vi "wrapper.vi"() -> ()   [LabVIEW 2016]
uses:
  QSM-PC (String)/Library/QSM-PC (String).lvlib
panel:
  out "控件值:QSM-Main":variant
  out "cluster_from main":cluster{"State":string, "Data":variant}
  out "cluster_\nsend to main":cluster{"State":string, "Data":variant}
  out "command":string
  out "ReadLine":string
  out "main_controls":cluster{"Name":string, "Variant Data":variant}[](array[cluster])
  out "QSM - wrapper":refnum<queue>
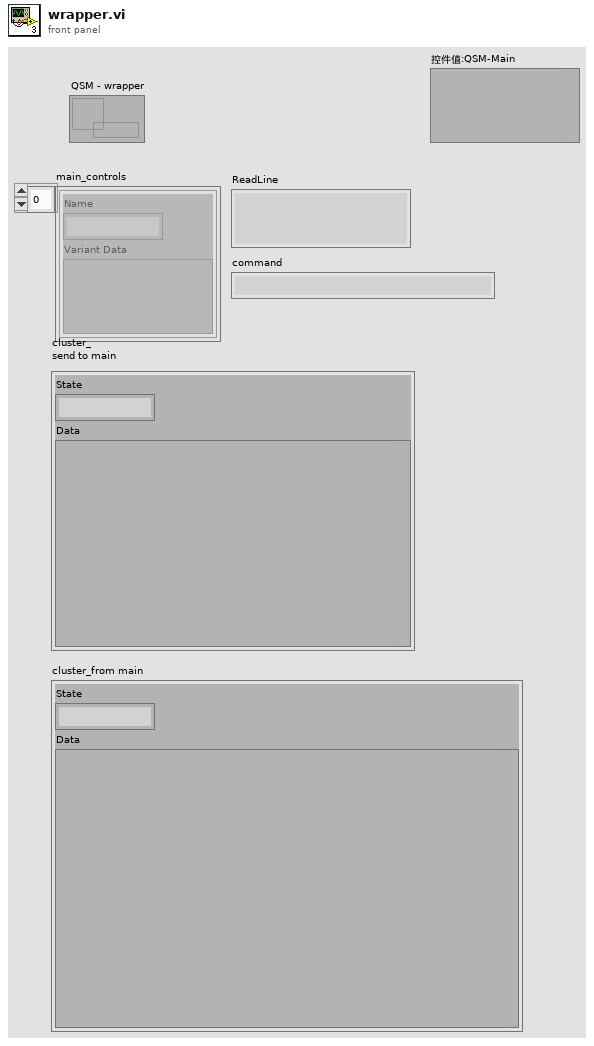
[diagram p1: front panel]
types:
  T1 = cluster{"app":string, "subject":string, "payload":cluster{"callback_msg":string}}
  T2 = cluster{"app":string, "subject":string, "payload":cluster{"callback_msg":dbl[][]}}
  T3 = cluster{"app":string, "subject":string, "payload":cluster{"time":string}}
  T4 = cluster{"app":string, "command":string, "payload":string}
  T5 = cluster{"app":string, "command":string, "payload":dbl}
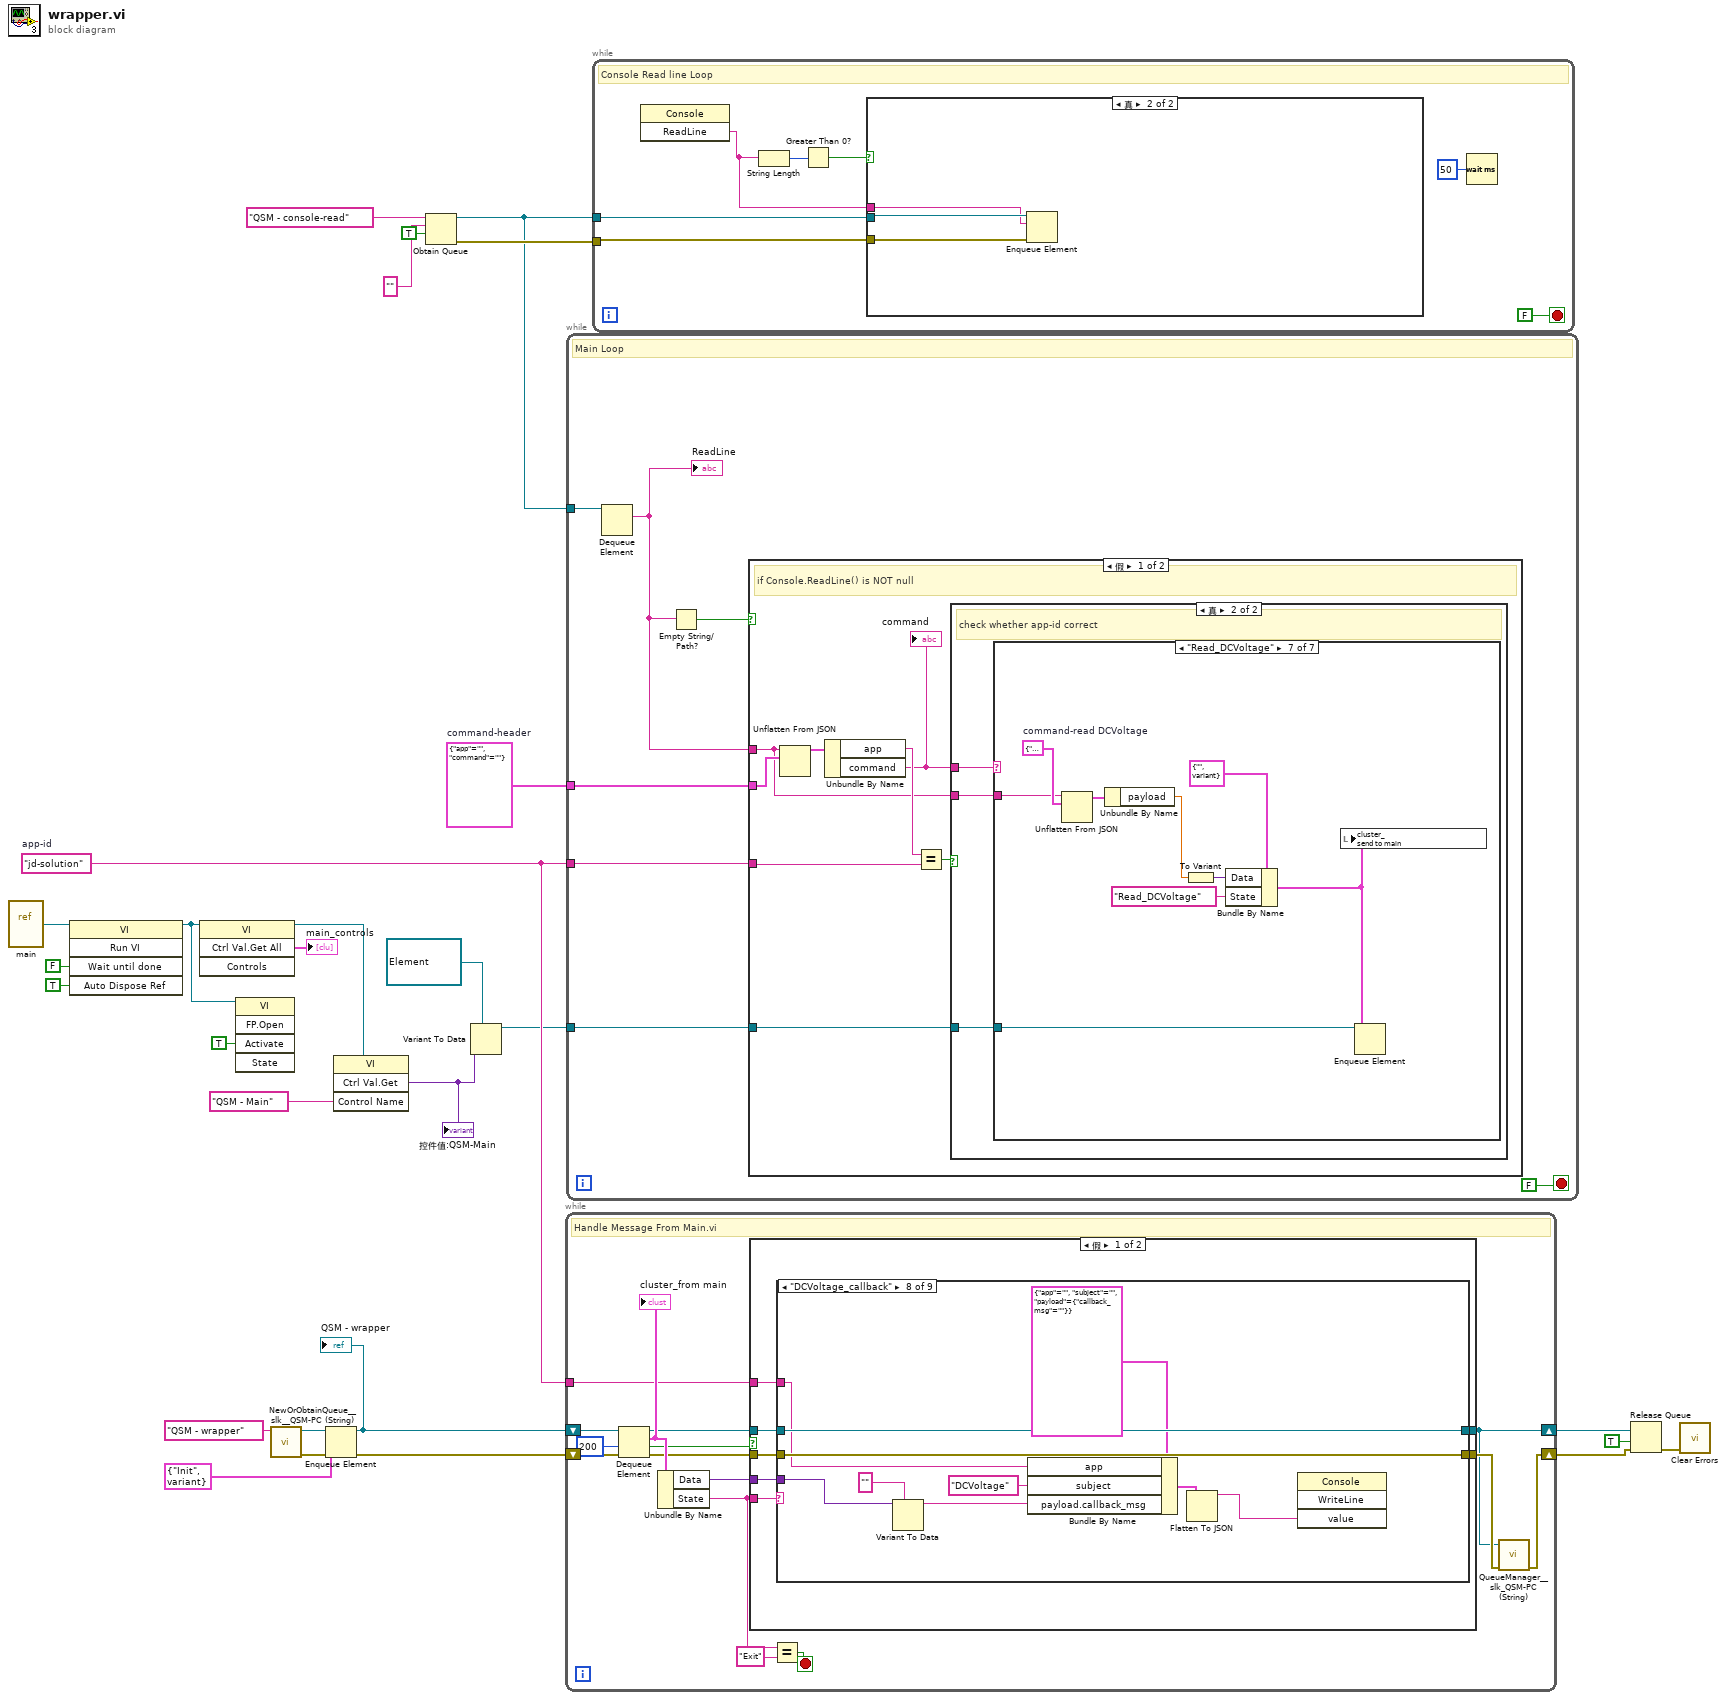
[diagram p0: block diagram]
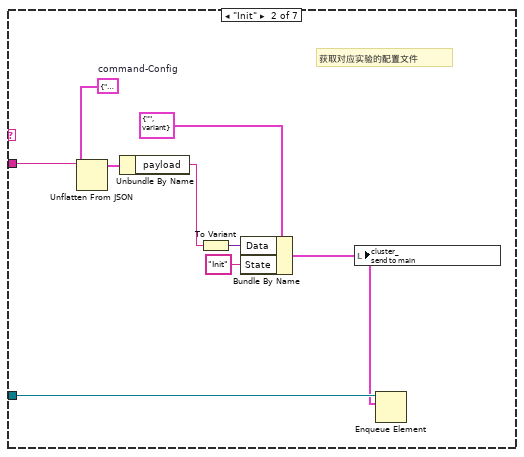
[diagram p5: hidden frame]
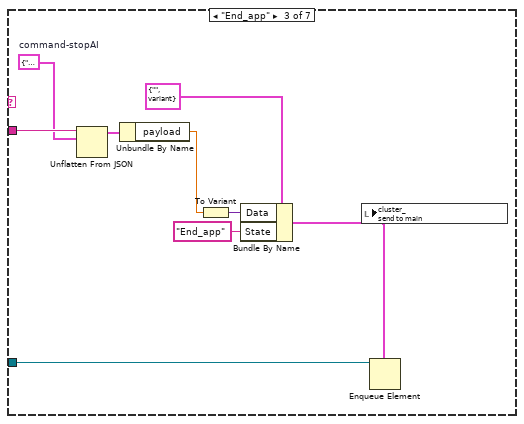
[diagram p6: hidden frame]
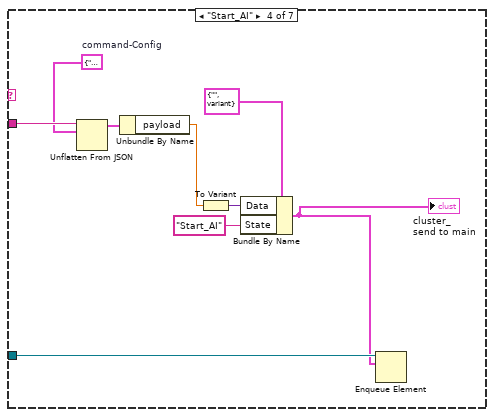
[diagram p7: hidden frame]
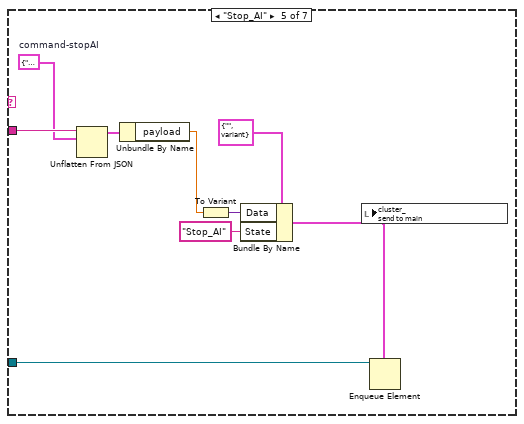
[diagram p8: hidden frame]
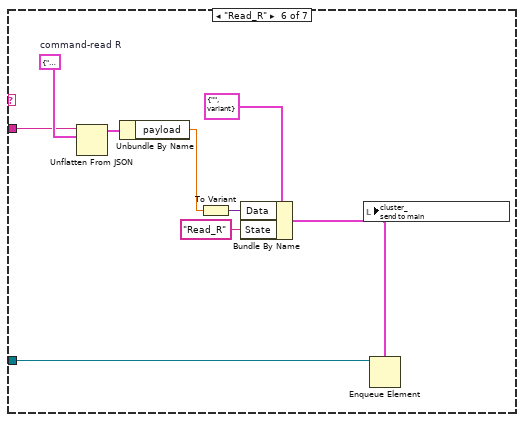
[diagram p9: hidden frame]
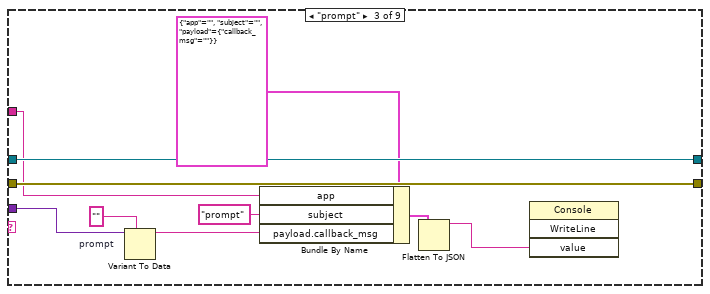
[diagram p13: hidden frame]
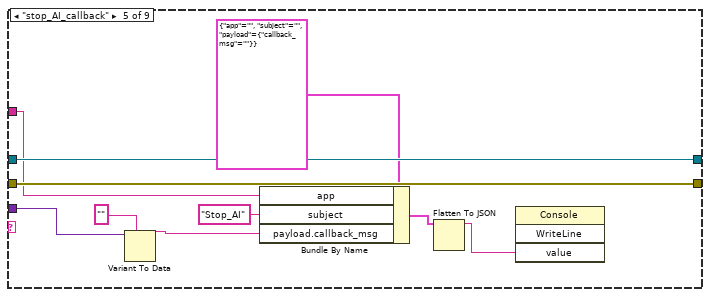
[diagram p15: hidden frame]
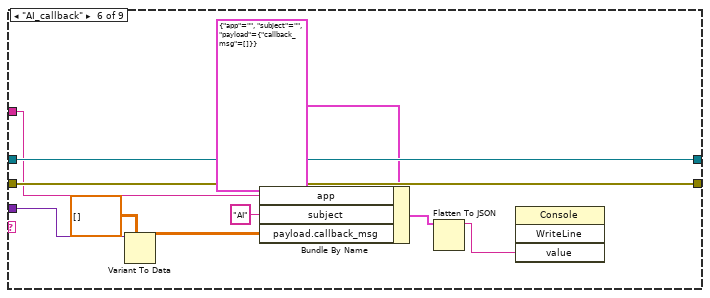
[diagram p16: hidden frame]
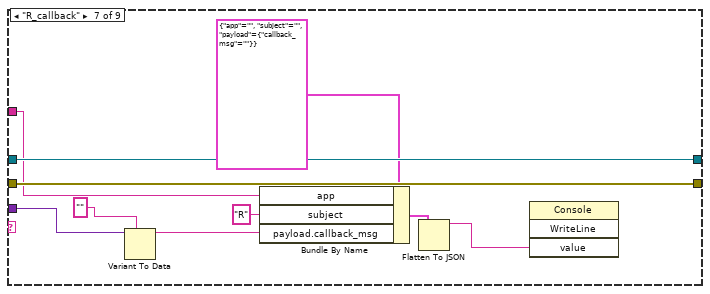
[diagram p17: hidden frame]
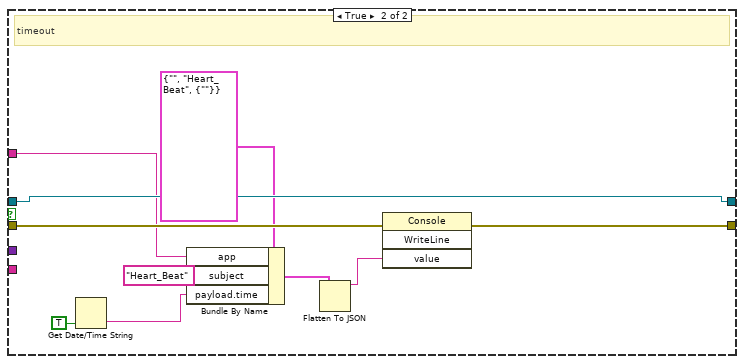
[diagram p19: hidden frame]
diagram:
  w9 = "jd-solution"  # app-id
  w10 = cluster{"app":string, "command":string} {"app"="", "command"=""}  # command-header
  n1 = vi-ref "main.vi"() -> (w15:refnum<vi>)
  n2 = invoke class="VI" method="Run VI"(reference=w15, "Wait until done"=FALSE ("结束前等待"), "Auto Dispose Ref"=TRUE ("自动销毁引用")) -> (reference out=w7:refnum<vi>)  [unwired: 2 in, 4 out]
  n3 = invoke class="VI" method="Ctrl Val.Get All"(reference=w7) -> (reference out=w12:refnum<vi>, "Get All Control Values Variant"=→"main_controls":cluster{"Name":string, "Variant Data":variant}[])  [unwired: 3 in, 2 out]
  n4 = invoke class="VI" method="FP.Open"(reference=w7, "Activate"=TRUE ("激活？")) -> ()  [unwired: 3 in, 5 out]
  n5 = call "NewOrObtainQueue__slk__QSM-PC (String).vi"("queue name in"="QSM - wrapper" ("name (unnamed)")) -> ("error out"=w25:errorcluster, "queue out"=w26:refnum<queue>)  [unwired: 2 in, 7 out]
  n6 = Enqueue Element(queue=w26, element=cluster{"State":string, "Data":variant} {"State"="Init", "Data"=variant} ("Element"), error in (no error)=w25) -> (queue out=w21:refnum<queue>, error out=w22:errorcluster)  [unwired: 2 out]
  "QSM - wrapper" <- w21
  n7 = invoke class="VI" method="Ctrl Val.Get"(reference=w12, "Control Name"="QSM - Main" ("控件名")) -> ("Get Control Value Variant"=w16:variant)  [unwired: 2 in, 3 out]
  "控件值:QSM-Main" <- w16
  n8 = Obtain Queue(name (unnamed)="QSM - console-read", element data type="", create if not found? (T)=TRUE ("如未找到则创建？(T)")) -> (queue out=w1:refnum<queue>, error out=w2:errorcluster)  [unwired: 2 in, 1 out]
  n9 = Variant To Data(type=refnum<queue> refnum ("队列输出"), Variant=w16) -> (data=w8:refnum<queue>)  [unwired: 1 in, 1 out]
  n10 = while {
    shift-right: [w34] -> w23
    shift-left: w21 -> [w43]
    shift-right: [w36] -> w20
    shift-left: w22 -> [w38]
    tunnel: w9 -> [w32]
    stop <- w33 stop-if-true
    # "Handle Message From Main.vi"
    n11 = Dequeue Element(queue=w43, timeout in ms (-1)=200 ("超时毫秒(-1)"), error in (no error)=w38) -> (queue out=w35:refnum<queue>, element=w42:cluster{"State":string, "Data":variant}, timed out?=w30:bool, error out=w37:errorcluster)
    "cluster_from main" <- w42
    n12 = Unbundle By Name(w42) -> ("Data"=w41:variant, "State"=w29:string)
    n13 = case shown="假" w30 {
      tunnel: w41 -> [w50 _]
      tunnel: w29 -> [w49 _]
      tunnel: [w48 w117] -> w39
      tunnel: w37 -> [w47 w118]
      tunnel: w35 -> [w46 w116]
      tunnel: [w45 w116] -> w34
      tunnel: w32 -> [w44 w113]
      frame False {
        n14 = case shown="\"DCVoltage_callback\"" w49 {
          tunnel: w50 -> [_ _ w62 _ w74 w84 w94 w104 _]
          tunnel: w47 -> [w51 w54 w63 w65 w75 w85 w95 w105 w108]
          tunnel: [w51 w54 w63 w65 w75 w85 w95 w105 w108] -> w48
          tunnel: w46 -> [w52 w53 w64 w66 w76 w86 w96 w106 w107]
          tunnel: [w52 w53 w64 w66 w76 w86 w96 w106 w107] -> w45
          tunnel: w44 -> [_ _ w58 _ w70 w80 w89 w100 _]
          frame "Idle", Default {
          }
          frame "Init" {
          }
          frame "prompt" {
            w57 = ""  # prompt
            n15 = Variant To Data(type=w57, Variant=w62) -> (data=w56:string)  [unwired: 1 in, 1 out]
            n16 = Bundle By Name(cluster=T1 {"app"="", "subject"="", "payload"={"callback_msg"=""}}, "app"=w58, "subject"="prompt", "payload.callback_msg"=w56) -> (w60:T1)
            n17 = Flatten To JSON(anything=w60) -> (JSON string=w55:string)  [unwired: 2 in, 1 out]
            n18 = invoke on="调用节点" class="Console" method="WriteLine"("value"=w55) -> ()  [unwired: 3 in, 4 out]
          }
          frame "Error_Handling" {
          }
          frame "stop_AI_callback" {
            n19 = Variant To Data(type="", Variant=w74) -> (data=w68:string)  [unwired: 1 in, 1 out]
            n20 = Bundle By Name(cluster=T1 {"app"="", "subject"="", "payload"={"callback_msg"=""}}, "app"=w70, "subject"="Stop_AI", "payload.callback_msg"=w68) -> (w72:T1)
            n21 = Flatten To JSON(anything=w72) -> (JSON string=w67:string)  [unwired: 2 in, 1 out]
            n22 = invoke on="调用节点" class="Console" method="WriteLine"("value"=w67) -> ()  [unwired: 3 in, 4 out]
          }
          frame "AI_callback" {
            n23 = Variant To Data(type=dbl[][] [], Variant=w84) -> (data=w78:dbl[][])  [unwired: 1 in, 1 out]
            n24 = Bundle By Name(cluster=T2 {"app"="", "subject"="", "payload"={"callback_msg"=[]}}, "app"=w80, "subject"="AI", "payload.callback_msg"=w78) -> (w82:T2)
            n25 = Flatten To JSON(anything=w82) -> (JSON string=w77:string)  [unwired: 2 in, 1 out]
            n26 = invoke on="调用节点" class="Console" method="WriteLine"("value"=w77) -> ()  [unwired: 3 in, 4 out]
          }
          frame "R_callback" {
            n27 = Variant To Data(type="", Variant=w94) -> (data=w87:string)  [unwired: 1 in, 1 out]
            n28 = Bundle By Name(cluster=T1 {"app"="", "subject"="", "payload"={"callback_msg"=""}}, "app"=w89, "subject"="R", "payload.callback_msg"=w87) -> (w92:T1)
            n29 = Flatten To JSON(anything=w92) -> (JSON string=w91:string)  [unwired: 2 in, 1 out]
            n30 = invoke on="调用节点" class="Console" method="WriteLine"("value"=w91) -> ()  [unwired: 3 in, 4 out]
          }
          frame "DCVoltage_callback" {
            n31 = Variant To Data(type="", Variant=w104) -> (data=w97:string)  [unwired: 1 in, 1 out]
            n32 = Bundle By Name(cluster=T1 {"app"="", "subject"="", "payload"={"callback_msg"=""}}, "app"=w100, "subject"="DCVoltage", "payload.callback_msg"=w97) -> (w103:T1)
            n33 = Flatten To JSON(anything=w103) -> (JSON string=w102:string)  [unwired: 2 in, 1 out]
            n34 = invoke on="调用节点" class="Console" method="WriteLine"("value"=w102) -> ()  [unwired: 3 in, 4 out]
          }
          frame "Exit" {
          }
        }
      }
      frame True {
        # "timeout"
        n35 = Get Date/Time String(want seconds? (F)=TRUE ("需要秒？(F)")) -> (time string=w110:string)  [unwired: 2 in, 1 out]
        n36 = Bundle By Name(cluster=T3 {"app"="", "subject"="Heart_Beat", "payload"={"time"=""}}, "app"=w113, "subject"="Heart_Beat", "payload.time"=w110) -> (w115:T3)
        n37 = Flatten To JSON(anything=w115) -> (JSON string=w111:string)  [unwired: 2 in, 1 out]
        n38 = invoke on="调用节点" class="Console" method="WriteLine"(error in=w118, "value"=w111) -> (error out=w117:errorcluster)  [unwired: 2 in, 3 out]
      }
    }
    n39 = Equal?(x=w29, y="Exit") -> (x = y?=w33:bool)
    n40 = call "QueueManager__slk_QSM-PC (String).vi"("queue in"=w34, "error in (no error)"=w39) -> ("error out"=w36:errorcluster)  [unwired: 2 in, 7 out]
  }
  n41 = while {
    tunnel: w10 -> [w124]
    tunnel: w9 -> [w123]
    tunnel: w8 -> [w122]
    tunnel: w1 -> [w120]
    stop <- FALSE stop-if-true
    # "Main Loop"
    n42 = Dequeue Element(queue=w120) -> (element=w119:string)  [unwired: 2 in, 3 out]
    "ReadLine" <- w119
    n43 = Empty String/Path?(string/path=w119) -> (empty?=w125:bool)
    n44 = case shown="假" w125 {
      tunnel: w119 -> [w127 _]
      tunnel: w124 -> [w133 _]
      tunnel: w123 -> [w129 _]
      tunnel: w122 -> [w126 _]
      frame False {
        # "if Console.ReadLine() is NOT null"
        n45 = Unflatten From JSON(JSON string=w127, type and defaults=w133) -> (value=w132:cluster{"app":string, "command":string})  [unwired: 5 in, 1 out]
        n46 = Unbundle By Name(w132) -> ("app"=w130:string, "command"=w128:string)
        "command" <- w128
        n47 = Equal?(x=w130, y=w129) -> (x = y?=w131:bool)
        n48 = case shown="真" w131 {
          tunnel: w128 -> [_ w136]
          tunnel: w127 -> [_ w135]
          tunnel: w126 -> [_ w134]
          frame False {
          }
          frame True {
            # "check whether app-id correct"
            n49 = case shown="\"Read_DCVoltage\"" w136 {
              tunnel: w135 -> [_ w145 w154 w163 w172 w174 w183]
              tunnel: w134 -> [_ w141 w150 w159 w168 w178 w187]
              frame "Idle", Default {
              }
              frame "Init" {
                w144 = T4 {"app"="", "command"="", "payload"="0"}  # command-Config
                # "获取对应实验的配置文件"
                n50 = Unflatten From JSON(JSON string=w145, type and defaults=w144) -> (value=w143:T4)  [unwired: 5 in, 1 out]
                n51 = Unbundle By Name(w143) -> ("payload"=w140:string)
                n52 = To Variant(anything=w140) -> (Variant=w142:variant)
                n53 = Bundle By Name(cluster=cluster{"State":string, "Data":variant} {"State"="", "Data"=variant} ("Element"), "Data"=w142, "State"="Init") -> (w138:cluster{"State":string, "Data":variant})
                n54 = local write "cluster_\nsend to main"(w138) -> ()
                n55 = Enqueue Element(queue=w141, element=w138) -> ()  [unwired: 2 in, 3 out]
              }
              frame "End_app" {
                w153 = T5 {"app"="", "command"="", "payload"=0.0}  # command-stopAI
                n56 = Unflatten From JSON(JSON string=w154, type and defaults=w153) -> (value=w152:T5)  [unwired: 5 in, 1 out]
                n57 = Unbundle By Name(w152) -> ("payload"=w149:dbl)
                n58 = To Variant(anything=w149) -> (Variant=w151:variant)
                n59 = Bundle By Name(cluster=cluster{"State":string, "Data":variant} {"State"="", "Data"=variant} ("Element"), "Data"=w151, "State"="End_app") -> (w147:cluster{"State":string, "Data":variant})
                n60 = local write "cluster_\nsend to main"(w147) -> ()
                n61 = Enqueue Element(queue=w150, element=w147) -> ()  [unwired: 2 in, 3 out]
              }
              frame "Start_AI" {
                w162 = T5 {"app"="", "command"="", "payload"=0.0}  # command-Config
                n62 = Unflatten From JSON(JSON string=w163, type and defaults=w162) -> (value=w161:T5)  [unwired: 5 in, 1 out]
                n63 = Unbundle By Name(w161) -> ("payload"=w155:dbl)
                n64 = To Variant(anything=w155) -> (Variant=w160:variant)
                n65 = Bundle By Name(cluster=cluster{"State":string, "Data":variant} {"State"="", "Data"=variant} ("Element"), "Data"=w160, "State"="Start_AI") -> (w158:cluster{"State":string, "Data":variant})
                "cluster_\nsend to main" <- w158
                n66 = Enqueue Element(queue=w159, element=w158) -> ()  [unwired: 2 in, 3 out]
              }
              frame "Stop_AI" {
                w171 = T5 {"app"="", "command"="", "payload"=0.0}  # command-stopAI
                n67 = Unflatten From JSON(JSON string=w172, type and defaults=w171) -> (value=w170:T5)  [unwired: 5 in, 1 out]
                n68 = Unbundle By Name(w170) -> ("payload"=w167:dbl)
                n69 = To Variant(anything=w167) -> (Variant=w169:variant)
                n70 = Bundle By Name(cluster=cluster{"State":string, "Data":variant} {"State"="", "Data"=variant} ("Element"), "Data"=w169, "State"="Stop_AI") -> (w166:cluster{"State":string, "Data":variant})
                n71 = local write "cluster_\nsend to main"(w166) -> ()
                n72 = Enqueue Element(queue=w168, element=w166) -> ()  [unwired: 2 in, 3 out]
              }
              frame "Read_R" {
                w181 = T5 {"app"="", "command"="", "payload"=0.0}  # command-read R
                n73 = Unflatten From JSON(JSON string=w174, type and defaults=w181) -> (value=w180:T5)  [unwired: 5 in, 1 out]
                n74 = Unbundle By Name(w180) -> ("payload"=w177:dbl)
                n75 = To Variant(anything=w177) -> (Variant=w179:variant)
                n76 = Bundle By Name(cluster=cluster{"State":string, "Data":variant} {"State"="", "Data"=variant} ("Element"), "Data"=w179, "State"="Read_R") -> (w175:cluster{"State":string, "Data":variant})
                n77 = local write "cluster_\nsend to main"(w175) -> ()
                n78 = Enqueue Element(queue=w178, element=w175) -> ()  [unwired: 2 in, 3 out]
              }
              frame "Read_DCVoltage" {
                w190 = T5 {"app"="", "command"="", "payload"=0.0}  # command-read DCVoltage
                n79 = Unflatten From JSON(JSON string=w183, type and defaults=w190) -> (value=w189:T5)  [unwired: 5 in, 1 out]
                n80 = Unbundle By Name(w189) -> ("payload"=w186:dbl)
                n81 = To Variant(anything=w186) -> (Variant=w188:variant)
                n82 = Bundle By Name(cluster=cluster{"State":string, "Data":variant} {"State"="", "Data"=variant} ("Element"), "Data"=w188, "State"="Read_DCVoltage") -> (w184:cluster{"State":string, "Data":variant})
                n83 = local write "cluster_\nsend to main"(w184) -> ()
                n84 = Enqueue Element(queue=w187, element=w184) -> ()  [unwired: 2 in, 3 out]
              }
            }
          }
        }
      }
      frame True {
        # "if Console.ReadLine() is  null"
      }
    }
  }
  n85 = while {
    tunnel: w1 -> [w193]
    tunnel: w2 -> [w191]
    stop <- FALSE stop-if-true
    # "Console Read line Loop"
    n86 = invoke on="调用节点" class="Console" method="ReadLine"() -> ("ReadLine"=w192:string)  [unwired: 3 in, 2 out]
    n87 = String Length(string=w192) -> (length=w195:i32)
    n88 = Greater Than 0?(x=w195) -> (x > 0?=w194:bool)
    n89 = case shown="真" w194 {
      tunnel: w193 -> [_ w200]
      tunnel: w192 -> [_ w199]
      tunnel: w191 -> [_ w198]
      frame False {
      }
      frame True {
        n90 = Enqueue Element(queue=w200, element=w199, error in (no error)=w198) -> ()  [unwired: 1 in, 3 out]
      }
    }
    n91 = Wait (ms)(milliseconds to wait=u32 50 ("等待时间（毫秒）")) -> ()  [unwired: 1 out]
  }
  n92 = Release Queue(queue=w23, force destroy? (F)=TRUE, error in (no error)=w20) -> (error out=w19:errorcluster)  [unwired: 2 out]
  n93 = call <vilib>:"Clear Errors.vi"("error in (no error)"=w19) -> ()  [unwired: 5 in, 2 out]
